vi "CreatePrivateEvents.vi"(8 "error in (no error)":errorcluster, 11 "Camera":refnum<class "Camera.lvclass">) -> (0 "error out":errorcluster, 3 "Camera out":refnum<class "Camera.lvclass">)   [LabVIEW 2015, in "Camera.lvclass"]
doc: "JKI State Machine Objects (SMO) 1.0.2.13\nJKI - JKI\nCopyright (c) 2016, JKI"
uses:
  Camera.lvclass
  Camera.lvclass/Camera.ctl
  Typedefs/PrivateEvents--Camera.Snap Image.ctl
  Typedefs/PrivateEvents--Camera.Save Image.ctl
  Typedefs/PrivateEvents--Camera.Get Image.ctl
  <vilib>/JKI/JKI SMO/SMO/SMO.lvclass
panel:
  # "For instructions on how to use the JKI State Machine Objects, examples and video tutorials, visit:\nhttp://jki.net/state-machine-objects/\n\nJKI State Machine Objects™\nhttp://jki.net/state-machine-objects/\nCopyright (C) 2005-2015, JKI <info@jki.net>\nALL RIGHTS RESERVED"
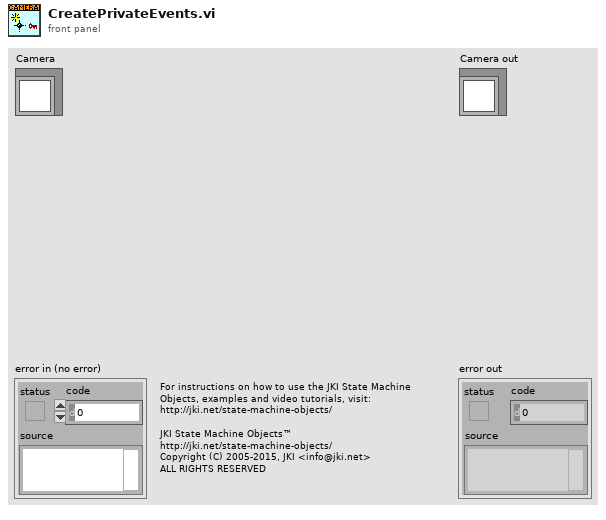
[diagram p1: front panel]
types:
  T1 = typedef "Camera.lvclass/PrivateData--Ref.ctl" = refnum<data-value>
  T2 = typedef "Camera.lvclass/PrivateEvents--Camera.Get Image.ctl" = i32
  T3 = typedef "Camera.lvclass/PrivateEvents--Camera.Save Image.ctl" = cluster{"Path":path, "index (-1: latest)":i32}
  T4 = typedef "Camera.lvclass/PrivateEvents--Camera.Snap Image.ctl" = refnum<notifier>
  T5 = typedef "Camera.lvclass/PrivateData--Cluster.ctl" = cluster{"Public Events":T6, "Protected Events":T7, "Private Events":T8, "Dependencies":T9}
  T6 = typedef "Camera.lvclass/PublicEvents--Cluster.ctl" = cluster{"NewImage":refnum<user-event>, "ImageSaved":refnum<user-event>}
  T7 = typedef "Camera.lvclass/ProtectedEvents--Cluster.ctl" = cluster{"placeholder":refnum<user-event>}
  T8 = typedef "Camera.lvclass/PrivateEvents--Cluster.ctl" = cluster{"Snap Image":refnum<user-event>, "Save Image":refnum<user-event>, "Get Image":refnum<user-event>}
  T9 = typedef "Camera.Simulated.lvclass/Dependencies--Cluster.ctl" = cluster{"CircularBuffer.ImageData":refnum<class "CircularBuffer.ImageData.lvclass">}
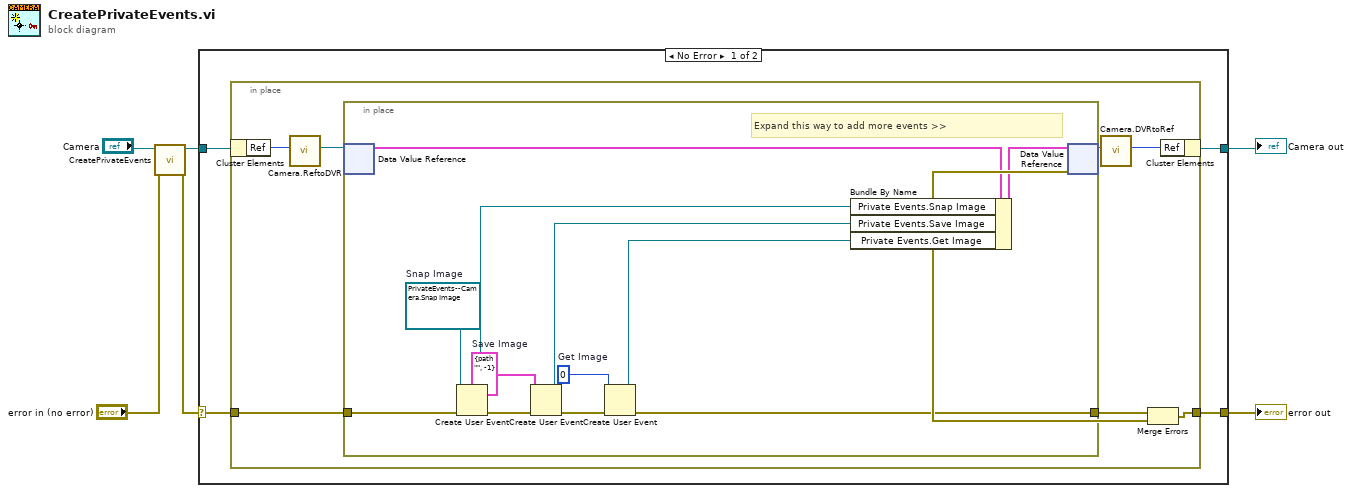
[diagram p0: block diagram]
diagram:
  n1 = call-parent "CreatePrivateEvents.vi"("error in (no error)"="error in (no error)", "SMO"="Camera") -> ("error out"=w5:errorcluster, "SMO out"=w6:refnum<class "Camera.lvclass">)  [unwired: 8 in]
  n2 = case shown="No Error" w5 {
    selector: w5 -> [w8 w32]
    tunnel: [w7 w32] -> w1
    tunnel: [w9 w31] -> w3
    tunnel: w6 -> [w10 w31]
    frame No Error {
      n3 = in-place {
        in-place-border: w8 -> [w18]
        in-place-border: [w15] -> w7
        n4 = in-place-cluster #1(w10) -> ("Ref"=w14:u32)
        n5 = call "Camera.ReftoDVR.vi"("Ref"=w14) -> ("Ref"=w13:T1)  [unwired: 10 in]
        n6 = in-place {
          in-place-border: w18 -> [w19]
          in-place-border: [w22] -> w17
          w21 = T2 0  # Get Image
          w24 = T3 {"Path"=path "", "index (-1: latest)"=-1}  # Save Image
          w27 = T4 refnum  # Snap Image
          # "Expand this way to add more events >>"
          n7 = in-place-dvr #2(w13) -> (w29:T5)  [unwired: 1 out]
          n8 = Create User Event(user event datatype=w27, error in=w19) -> (user event=w26:refnum<user-event>, error out=w28:errorcluster)
          n9 = Create User Event(user event datatype=w24, error in=w28) -> (user event=w23:refnum<user-event>, error out=w25:errorcluster)
          n10 = Create User Event(user event datatype=w21, error in=w25) -> (user event=w20:refnum<user-event>, error out=w22:errorcluster)
          n11 = Bundle By Name(cluster=w29, "Private Events.Snap Image"=w26, "Private Events.Save Image"=w23, "Private Events.Get Image"=w20) -> (w30:T5)
          n12 = in-place-dvr #2(w30) -> (w12:T1, w16:errorcluster)
        }
        n13 = call "Camera.DVRtoRef.vi"("Ref"=w12) -> ("Ref"=w11:u32)  [unwired: 10 in]
        n14 = Merge Errors(w17, w16) -> (w15:errorcluster)
        n15 = in-place-cluster #1("Ref"=w11) -> (w9:refnum<class "Camera.lvclass">)
      }
    }
    frame Error {
    }
  }
  "error out" <- w1
  "Camera out" <- w3
